vi "rsscope_core_global.vi"() -> ()   [LabVIEW 2018] (continued)
TrigA, TrigB, TrigR\r\n\nRemote-control command(s):\nTRIGger<m>:RFFE:ERRor:USEQuence"}, {"Level"=4, "Class Only"=FALSE, "Identifier"="RSSCOPE_ATTR_PROTOCOL_RFFE_TRIGGER_ERROR_GAP", "Descriptive Name"="Protocol RFFE Trigger Error Gap", "Data Type"=3, "Command"="TRIG{Trigger}:RFFE:ERR:GAP", "Access"=2, "Range Table"="", "Read Callback"="", "Write Callback"="", "Supported Models"="", "Instrument Options"="K40", "Flags"=0, "Help"="Enables the trigger on a gap error.\n\nAvailable Repeated Capabilities:\nTrigger: TrigA, TrigB, TrigR\r\n\nRemote-control command(s):\nTRIGger<m>:RFFE:ERRor:GAP"}, {"Level"=4, "Class Only"=FALSE, "Identifier"="RSSCOPE_ATTR_PROTOCOL_RFFE_TRIGGER_ERROR_VERSION", "Descriptive Name"="Protocol RFFE Trigger Error Version", "Data Type"=3, "Command"="TRIG{Trigger}:RFFE:ERR:VERS", "Access"=2, "Range Table"="", "Read Callback"="", "Write Callback"="", "Supported Models"="", "Instrument Options"="K40", "Flags"=0, "Help"="Enables the trigger on RFFE version error.\n\nAvailable Repeated Capabilities:\nTrigger: TrigA, TrigB, TrigR\r\n\nRemote-control command(s):\nTRIGger<m>:RFFE:ERRor:VERSion"}, {"Level"=2, "Class Only"=TRUE, "Identifier"="", "Descriptive Name"="MDIO", "Data Type"=0, "Command"="", "Access"=0, "Range Table"="", "Read Callback"="", "Write Callback"="", "Supported Models"="", "Instrument Options"="", "Flags"=0, "Help"="Configures MDIO trigger, option K55."}, {"Level"=3, "Class Only"=FALSE, "Identifier"="RSSCOPE_ATTR_PROTOCOL_MDIO_TRIGGER_TYPE", "Descriptive Name"="Protocol MDIO Trigger Type", "Data Type"=0, "Command"="TRIG{Trigger}:MDIO:TYPE", "Access"=2, "Range Table"="rsscope_rngProtocolMDIOTriggerType", "Read Callback"="", "Write Callback"="", "Supported Models"="", "Instrument Options"="K55", "Flags"=0, "Help"="Selects the trigger type for MDIO analysis.\n\nAvailable Repeated Capabilities:\nTrigger: TrigA, TrigB, TrigR\r\n\nRemote-control command(s):\nTRIGger<m>:MDIO:TYPE"}, {"Level"=3, "Class Only"=FALSE, "Identifier"="RSSCOPE_ATTR_PROTOCOL_MDIO_TRIGGER_START_CODE", "Descriptive Name"="Protocol MDIO Trigger Start Code", "Data Type"=0, "Command"="TRIG{Trigger}:MDIO:ST", "Access"=2, "Range Table"="rsscope_rngProtocolMDIOTriggerStartCode", "Read Callback"="", "Write Callback"="", "Supported Models"="", "Instrument Options"="K55", "Flags"=0, "Help"="Selects the start of frame code of the frame pattern.\n\nAvailable Repeated Capabilities:\nTrigger: TrigA, TrigB, TrigR\r\n\nRemote-control command(s):\nTRIGger<m>:MDIO:ST"}, {"Level"=3, "Class Only"=FALSE, "Identifier"="RSSCOPE_ATTR_PROTOCOL_MDIO_TRIGGER_OPERATION_CODE", "Descriptive Name"="Protocol MDIO Trigger Operation Code", "Data Type"=0, "Command"="TRIG{Trigger}:MDIO:FRAM", "Access"=2, "Range Table"="rsscope_rngProtocolMDIOTriggerOperationCode", "Read Callback"="", "Write Callback"="", "Supported Models"="", "Instrument Options"="K55", "Flags"=0, "Help"="Selects the Type of Frame code (or OP code, OpCode, operation code).\n\nAvailable Repeated Capabilities:\nTrigger: TrigA, TrigB, TrigR\r\n\nRemote-control command(s):\nTRIGger<m>:MDIO:FRAMetype"}, {"Level"=3, "Class Only"=FALSE, "Identifier"="RSSCOPE_ATTR_PROTOCOL_MDIO_TRIGGER_PHYSICAL_PORT_ADDRESS", "Descriptive Name"="Protocol MDIO Trigger Physical Port Address", "Data Type"=2, "Command"="TRIG{Trigger}:MDIO:PHYS", "Access"=2, "Range Table"="", "Read Callback"="", "Write Callback"="", "Supported Models"="", "Instrument Options"="K55", "Flags"=0, "Help"="Sets the physical address (in Clause 22) or port address (in Clause 45) of the frame pattern (5 bits).\n\nAvailable Repeated Capabilities:\nTrigger: TrigA, TrigB, TrigR\r\n\nRemote-control command(s):\nTRIGger<m>:MDIO:PHYS"}, {"Level"=3, "Class Only"=FALSE, "Identifier"="RSSCOPE_ATTR_PROTOCOL_MDIO_TRIGGER_REGISTER_DEVICE_ADDRESS", "Descriptive Name"="Protocol MDIO Trigger Register Device Address", "Data Type"=2, "Command"="TRIG{Trigger}:MDIO:REGI", "Access"=2, "Range Table"="", "Read Callback"="", "Write Callback"="", "Supported Models"="", "Instrument Options"="K55", "Flags"=0, "Help"="Sets the register address (in Clause 22) or device address (in Clause 45) of the frame pattern (5 bits); available only in trigger type &apos;Data&apos;.\n\nAvailable Repeated Capabilities:\nTrigger: TrigA, TrigB, TrigR\r\n\nRemote-control command(s):\nTRIGger<m>:MDIO:REGI"}, {"Level"=3, "Class Only"=FALSE, "Identifier"="RSSCOPE_ATTR_PROTOCOL_MDIO_TRIGGER_DATA_ADDRESS_PATTERN", "Descriptive Name"="Protocol MDIO Trigger Data Address Pattern", "Data Type"=2, "Command"="TRIG{Trigger}:MDIO:DATA", "Access"=2, "Range Table"="", "Read Callback"="", "Write Callback"="", "Supported Models"="", "Instrument Options"="K55", "Flags"=0, "Help"="Defines the 16-bit payload data pattern (both in Clause 22 or Clause 45) or the address pattern (in Clause 45, only) to trigger for.\n\nAvailable Repeated Capabilities:\nTrigger: TrigA, TrigB, TrigR\r\n\nRemote-control command(s):\nTRIGger<m>:MDIO:DATA"}, {"Level"=2, "Class Only"=TRUE, "Identifier"="", "Descriptive Name"="Ethernet", "Data Type"=0, "Command"="", "Access"=0, "Range Table"="", "Read Callback"="", "Write Callback"="", "Supported Models"="", "Instrument Options"="", "Flags"=0, "Help"="Configures Ethernet trigger settings.\n\nAttributes in this class require option R&S RTO-K8."}, {"Level"=3, "Class Only"=FALSE, "Identifier"="RSSCOPE_ATTR_ETHERNET_TRIGGER_TYPE", "Descriptive Name"="Ethernet Trigger Type", "Data Type"=0, "Command"="TRIG{Trigger}:ETH:TYPE", "Access"=2, "Range Table"="RsScope_rngEthernetTriggerType", "Read Callback"="", "Write Callback"="", "Supported Models"="", "Instrument Options"="K8", "Flags"=0, "Help"="Sets the trigger type for Ethernet variant 10BASE-T.\n\nAvailable Repeated Capabilities:\nTrigger: TrigA, TrigB, TrigR\r\n\nRemote-control command(s):\nTRIGger<m>:ETHernet:TYPE"}, {"Level"=3, "Class Only"=FALSE, "Identifier"="RSSCOPE_ATTR_ETHERNET_TRIGGER_PATTERN", "Descriptive Name"="Ethernet Trigger Pattern", "Data Type"=2, "Command"="TRIG{Trigger}:ETH:PATT", "Access"=2, "Range Table"="", "Read Callback"="", "Write Callback"="", "Supported Models"="", "Instrument Options"="K8", "Flags"=0, "Help"="Specifies the bit pattern (or data) that is to be triggered.\n\nAvailable Repeated Capabilities:\nTrigger: TrigA, TrigB, TrigR\r\n\nRemote-control command(s):\nTRIGger<m>:ETHernet:PATTern"}, {"Level"=3, "Class Only"=FALSE, "Identifier"="RSSCOPE_ATTR_ETHERNET_TRIGGER_ERROR_CRC", "Descriptive Name"="Ethernet Trigger Error CRC", "Data Type"=3, "Command"="TRIG{Trigger}:ETH:ERR:CRC", "Access"=2, "Range Table"="", "Read Callback"="", "Write Callback"="", "Supported Models"="", "Instrument Options"="K8", "Flags"=0, "Help"="Enables the trigger on a mismatch of the cyclic redundancy check (CRC) value between the transmitting and receiving device.\n\nAvailable Repeated Capabilities:\nTrigger: TrigA, TrigB, TrigR\r\n\nRemote-control command(s):\nTRIGger<m>:ETHernet:ERRor:CRC"}, {"Level"=3, "Class Only"=FALSE, "Identifier"="RSSCOPE_ATTR_ETHERNET_TRIGGER_ERROR_LENGTH", "Descriptive Name"="Ethernet Trigger Error Length", "Data Type"=3, "Command"="TRIG{Trigger}:ETH:ERR:LENG", "Access"=2, "Range Table"="", "Read Callback"="", "Write Callback"="", "Supported Models"="", "Instrument Options"="K8", "Flags"=0, "Help"="Enables the trigger on an incorrect length of the sequence - when additional or missing bits are detected and the sequence of bits is not as expected.\n\nAvailable Repeated Capabilities:\nTrigger: TrigA, TrigB, TrigR\r\n\nRemote-control command(s):\nTRIGger<m>:ETHernet:ERRor:LENGth"}, {"Level"=3, "Class Only"=FALSE, "Identifier"="RSSCOPE_ATTR_ETHERNET_TRIGGER_ERROR_PREAMBLE", "Descriptive Name"="Ethernet Trigger Error Preamble", "Data Type"=3, "Command"="TRIG{Trigger}:ETH:ERR:PRE", "Access"=2, "Range Table"="", "Read Callback"="", "Write Callback"="", "Supported Models"="", "Instrument Options"="K8", "Flags"=0, "Help"="Enables the trigger on a frame with invalid preamble.\n\nAvailable Repeated Capabilities:\nTrigger: TrigA, TrigB, TrigR\r\n\nRemote-control command(s):\nTRIGger<m>:ETHernet:ERRor:PREamble"}, {"Level"=3, "Class Only"=TRUE, "Identifier"="", "Descriptive Name"="Frame", "Data Type"=0, "Command"="", "Access"=0, "Range Table"="", "Read Callback"="", "Write Callback"="", "Supported Models"="", "Instrument Options"="", "Flags"=0, "Help"="Configures Ethernet frame."}, {"Level"=4, "Class Only"=FALSE, "Identifier"="RSSCOPE_ATTR_ETHERNET_TRIGGER_FRAME_CRC_CONDITION", "Descriptive Name"="Ethernet Trigger Frame CRC Condition", "Data Type"=0, "Command"="TRIG{Trigger}:ETH:FRAM:CCON", "Access"=2, "Range Table"="RsScope_rngProtocolEthernetTriggerDataCondition", "Read Callback"="", "Write Callback"="", "Supported Models"="", "Instrument Options"="K8", "Flags"=0, "Help"="Sets the operator to trigger on a specific frame check sequence value.\n\nAvailable Repeated Capabilities:\nTrigger: TrigA, TrigB, TrigR\r\n\nRemote-control command(s):\nTRIGger<m>:ETHernet:FRAMe:CCONdition"}, {"Level"=4, "Class Only"=FALSE, "Identifier"="RSSCOPE_ATTR_ETHERNET_TRIGGER_FRAME_CRC_PATTERN_MIN", "Descriptive Name"="Ethernet Trigger Frame CRC Pattern Min", "Data Type"=2, "Command"="TRIG{Trigger}:ETH:FRAM:CMIN", "Access"=2, "Range Table"="", "Read Callback"="", "Write Callback"="", "Supported Models"="", "Instrument Options"="K8", "Flags"=0, "Help"="Specifies a CRC pattern, or sets the start value of a pattern range.\n\nAvailable Repeated Capabilities:\nTrigger: TrigA, TrigB, TrigR\r\n\nRemote-control command(s):\nTRIGger<m>:ETHernet:FRAMe:CMIN"}, {"Level"=4, "Class Only"=FALSE, "Identifier"="RSSCOPE_ATTR_ETHERNET_TRIGGER_FRAME_CRC_PATTERN_MAX", "Descriptive Name"="Ethernet Trigger Frame CRC Pattern Max", "Data Type"=2, "Command"="TRIG{Trigger}:ETH:FRAM:CMAX", "Access"=2, "Range Table"="", "Read Callback"="", "Write Callback"="", "Supported Models"="", "Instrument Options"="K8", "Flags"=0, "Help"="Sets the end value of the frame check sequence range.\n\nAvailable Repeated Capabilities:\nTrigger: TrigA, TrigB, TrigR\r\n\nRemote-control command(s):\nTRIGger<m>:ETHernet:FRAMe:CMAX"}, {"Level"=4, "Class Only"=FALSE, "Identifier"="RSSCOPE_ATTR_ETHERNET_TRIGGER_FRAME_DESTINATION_ADDRESS_CONDITION", "Descriptive Name"="Ethernet Trigger Frame Destination Address Condition", "Data Type"=0, "Command"="TRIG{Trigger}:ETH:FRAM:DCON", "Access"=2, "Range Table"="RsScope_rngProtocolEthernetTriggerDataCondition", "Read Callback"="", "Write Callback"="", "Supported Models"="", "Instrument Options"="K8", "Flags"=0, "Help"="Sets the destination address operator to trigger on a specific pattern or a range.\n\nAvailable Repeated Capabilities:\nTrigger: TrigA, TrigB, TrigR\r\n\nRemote-control command(s):\nTRIGger<m>:ETHernet:FRAMe:DCONdition"}, {"Level"=4, "Class Only"=FALSE, "Identifier"="RSSCOPE_ATTR_ETHERNET_TRIGGER_FRAME_DESTINATION_ADDRESS_PATTERN_MIN", "Descriptive Name"="Ethernet Trigger Frame Destination Address Pattern Min", "Data Type"=2, "Command"="TRIG{Trigger}:ETH:FRAM:DMIN", "Access"=2, "Range Table"="", "Read Callback"="", "Write Callback"="", "Supported Models"="", "Instrument Options"="K8", "Flags"=0, "Help"="Specifies a destination address pattern, or sets the start value of a pattern range.\n\nAvailable Repeated Capabilities:\nTrigger: TrigA, TrigB, TrigR\r\n\nRemote-control command(s):\nTRIGger<m>:ETHernet:FRAMe:DMIN"}, {"Level"=4, "Class Only"=FALSE, "Identifier"="RSSCOPE_ATTR_ETHERNET_TRIGGER_FRAME_DESTINATION_ADDRESS_PATTERN_MAX", "Descriptive Name"="Ethernet Trigger Frame Destination Address Pattern Max", "Data Type"=2, "Command"="TRIG{Trigger}:ETH:FRAM:DMAX", "Access"=2, "Range Table"="", "Read Callback"="", "Write Callback"="", "Supported Models"="", "Instrument Options"="K8", "Flags"=0, "Help"="Sets the end value of a destination address range.\n\nAvailable Repeated Capabilities:\nTrigger: TrigA, TrigB, TrigR\r\n\nRemote-control command(s):\nTRIGger<m>:ETHernet:FRAMe:DMAX"}, {"Level"=4, "Class Only"=FALSE, "Identifier"="RSSCOPE_ATTR_ETHERNET_TRIGGER_FRAME_SOURCE_ADDRESS_CONDITION", "Descriptive Name"="Ethernet Trigger Frame Source Address Condition", "Data Type"=0, "Command"="TRIG{Trigger}:ETH:FRAM:SCON", "Access"=2, "Range Table"="RsScope_rngProtocolEthernetTriggerDataCondition", "Read Callback"="", "Write Callback"="", "Supported Models"="", "Instrument Options"="K8", "Flags"=0, "Help"="Sets source address operator to trigger on a specific pattern or a range.\n\nAvailable Repeated Capabilities:\nTrigger: TrigA, TrigB, TrigR\r\n\nRemote-control command(s):\nTRIGger<m>:ETHernet:FRAMe:SCONdition"}, {"Level"=4, "Class Only"=FALSE, "Identifier"="RSSCOPE_ATTR_ETHERNET_TRIGGER_FRAME_SOURCE_ADDRESS_PATTERN_MIN", "Descriptive Name"="Ethernet Trigger Frame Source Address Pattern Min", "Data Type"=2, "Command"="TRIG{Trigger}:ETH:FRAM:SMIN", "Access"=2, "Range Table"="", "Read Callback"="", "Write Callback"="", "Supported Models"="", "Instrument Options"="K8", "Flags"=0, "Help"="Specifies a source address pattern, or sets the start value of a pattern range.\n\nAvailable Repeated Capabilities:\nTrigger: TrigA, TrigB, TrigR\r\n\nRemote-control command(s):\nTRIGger<m>:ETHernet:FRAMe:SMIN"}, {"Level"=4, "Class Only"=FALSE, "Identifier"="RSSCOPE_ATTR_ETHERNET_TRIGGER_FRAME_SOURCE_ADDRESS_PATTERN_MAX", "Descriptive Name"="Ethernet Trigger Frame Source Address Pattern Max", "Data Type"=2, "Command"="TRIG{Trigger}:ETH:FRAM:SMAX", "Access"=2, "Range Table"="", "Read Callback"="", "Write Callback"="", "Supported Models"="", "Instrument Options"="K8", "Flags"=0, "Help"="Sets the end value of a source address range.\n\nAvailable Repeated Capabilities:\nTrigger: TrigA, TrigB, TrigR\r\n\nRemote-control command(s):\nTRIGger<m>:ETHernet:FRAMe:SMAX"}, {"Level"=4, "Class Only"=FALSE, "Identifier"="RSSCOPE_ATTR_ETHERNET_TRIGGER_FRAME_TYPE_OPERATOR_CONDITION", "Descriptive Name"="Ethernet Trigger Frame Type Operator Condition", "Data Type"=0, "Command"="TRIG{Trigger}:ETH:FRAM:TCON", "Access"=2, "Range Table"="RsScope_rngProtocolEthernetTriggerDataCondition", "Read Callback"="", "Write Callback"="", "Supported Models"="", "Instrument Options"="K8", "Flags"=0, "Help"="Sets the type operator to trigger on a specific length/type value pattern or a range.\n\nAvailable Repeated Capabilities:\nTrigger: TrigA, TrigB, TrigR\r\n\nRemote-control command(s):\nTRIGger<m>:ETHernet:FRAMe:TCONdition"}, {"Level"=4, "Class Only"=FALSE, "Identifier"="RSSCOPE_ATTR_ETHERNET_TRIGGER_FRAME_TYPE_OPERATOR_PATTERN_MIN", "Descriptive Name"="Ethernet Trigger Frame Type Operator Pattern Min", "Data Type"=2, "Command"="TRIG{Trigger}:ETH:FRAM:TMIN", "Access"=2, "Range Table"="", "Read Callback"="", "Write Callback"="", "Supported Models"="", "Instrument Options"="K8", "Flags"=0, "Help"="Specifies a length/type value, or sets the start value of a pattern range.\n\nAvailable Repeated Capabilities:\nTrigger: TrigA, TrigB, TrigR\r\n\nRemote-control command(s):\nTRIGger<m>:ETHernet:FRAMe:TMIN"}, {"Level"=4, "Class Only"=FALSE, "Identifier"="RSSCOPE_ATTR_ETHERNET_TRIGGER_FRAME_TYPE_OPERATOR_PATTERN_MAX", "Descriptive Name"="Ethernet Trigger Frame Type Operator Pattern Max", "Data Type"=2, "Command"="TRIG{Trigger}:ETH:FRAM:TMAX", "Access"=2, "Range Table"="", "Read Callback"="", "Write Callback"="", "Supported Models"="", "Instrument Options"="K8", "Flags"=0, "Help"="Sets the end value of a length/type range.\n\nAvailable Repeated Capabilities:\nTrigger: TrigA, TrigB, TrigR\r\n\nRemote-control command(s):\nTRIGger<m>:ETHernet:FRAMe:TMAX"}, {"Level"=2, "Class Only"=TRUE, "Identifier"="", "Descriptive Name"="USB", "Data Type"=0, "Command"="", "Access"=0, "Range Table"="", "Read Callback"="", "Write Callback"="", "Supported Models"="", "Instrument Options"="", "Flags"=0, "Help"="Configures USB trigger settings."}, {"Level"=3, "Class Only"=FALSE, "Identifier"="RSSCOPE_ATTR_PROTOCOL_USB_TRIGGER_TYPE", "Descriptive Name"="Protocol USB Trigger Type", "Data Type"=0, "Command"="TRIG{Trigger}:USB:TYPE", "Access"=2, "Range Table"="rsscope_rngProtocolUSBTriggerType", "Read Callback"="", "Write Callback"="", "Supported Models"="", "Instrument Options"="K60", "Flags"=0, "Help"="Selects the trigger type for USB analysis. The available trigger types depend on the activated USB protocol type.\n\nAvailable Repeated Capabilities:\nTrigger: TrigA, TrigB, TrigR\r\n\nRemote-control command(s):\nTRIGger<m>:USB:TYPE"}, {"Level"=3, "Class Only"=FALSE, "Identifier"="RSSCOPE_ATTR_PROTOCOL_USB_TRIGGER_TOKEN", "Descriptive Name"="Protocol USB Trigger Token", "Data Type"=0, "Command"="TRIG{Trigger}:USB:TOK", "Access"=2, "Range Table"="rsscope_rngProtocolUSBTriggerToken", "Read Callback"="", "Write Callback"="", "Supported Models"="", "Instrument Options"="K60", "Flags"=0, "Help"="Sets the trigger to one out of four different token types: Out, In, Start of Frame, or Setup.\n\nAvailable Repeated Capabilities:\nTrigger: TrigA, TrigB, TrigR\r\n\nRemote-control command(s):\nTRIGger<m>:USB:TOKen"}, {"Level"=3, "Class Only"=FALSE, "Identifier"="RSSCOPE_ATTR_PROTOCOL_USB_TRIGGER_DATA_TYPE", "Descriptive Name"="Protocol USB Trigger Data Type", "Data Type"=0, "Command"="TRIG{Trigger}:USB:DATA", "Access"=2, "Range Table"="rsscope_rngProtocolUSBTriggerDataType", "Read Callback"="", "Write Callback"="", "Supported Models"="", "Instrument Options"="K60", "Flags"=0, "Help"="Sets the trigger to one out of four different payload data types: DATA0, DATA1, DATA2, or MDATA.\n\nAvailable Repeated Capabilities:\nTrigger: TrigA, TrigB, TrigR\r\n\nRemote-control command(s):\nTRIGger<m>:USB:DATA"}, {"Level"=3, "Class Only"=FALSE, "Identifier"="RSSCOPE_ATTR_PROTOCOL_USB_TRIGGER_HANDSHAKE", "Descriptive Name"="Protocol USB Trigger Handshake", "Data Type"=0, "Command"="TRIG{Trigger}:USB:HAND", "Access"=2, "Range Table"="rsscope_rngProtocolUSBTriggerHandshake", "Read Callback"="", "Write Callback"="", "Supported Models"="", "Instrument Options"="", "Flags"=0, "Help"="Sets the trigger to one out of four different handshake types: acknowledgment, non-acknowledgment, stall, or no response.\n\nAvailable Repeated Capabilities:\nTrigger: TrigA, TrigB, TrigR\r\n\nRemote-control command(s):\nTRIGger<m>:USB:HAND"}, {"Level"=3, "Class Only"=FALSE, "Identifier"="RSSCOPE_ATTR_PROTOCOL_USB_TRIGGER_SPECIAL_PID", "Descriptive Name"="Protocol USB Trigger Special PID", "Data Type"=0, "Command"="TRIG{Trigger}:USB:SPEC", "Access"=2, "Range Table"="rsscope_rngProtocolUSBTriggerSpecialPID", "Read Callback"="", "Write Callback"="", "Supported Models"="", "Instrument Options"="K60", "Flags"=0, "Help"="Sets the trigger to one out of four different Special PID types: Preamble, Error, Split, or Ping.\n\nAvailable Repeated Capabilities:\nTrigger: TrigA, TrigB, TrigR\r\n\nRemote-control command(s):\nTRIGger<m>:USB:SPEC"}, {"Level"=3, "Class Only"=FALSE, "Identifier"="RSSCOPE_ATTR_PROTOCOL_USB_TRIGGER_ERROR_CONDITION", "Descriptive Name"="Protocol USB Trigger Error Condition", "Data Type"=0, "Command"="TRIG{Trigger}:USB:ERRC", "Access"=2, "Range Table"="rsscope_rngProtocolUSBTriggerErrorCondition", "Read Callback"="", "Write Callback"="", "Supported Models"="", "Instrument Options"="K60", "Flags"=0, "Help"="Sets the trigger to one of the following eight error condition types: PID error, CRC5 error, CRC16 error, Bitstuffing error, unexpected PID error, SE1 error, or Glitching error, as well as Any of these errors.\n\nAvailable Repeated Capabilities:\nTrigger: TrigA, TrigB, TrigR\r\n\nRemote-control command(s):\nTRIGger<m>:USB:ERRC"}, {"Level"=3, "Class Only"=FALSE, "Identifier"="RSSCOPE_ATTR_PROTOCOL_USB_TRIGGER_PID_ERROR_CHECK", "Descriptive Name"="Protocol USB Trigger PID Error Check", "Data Type"=3, "Command"="TRIG{Trigger}:USB:WPID", "Access"=2, "Range Table"="", "Read Callback"="", "Write Callback"="", "Supported Models"="", "Instrument Options"="K60", "Flags"=0, "Help"="Defines, whether the packet ID error check shall be activated or not.\n\nAvailable Repeated Capabilities:\nTrigger: TrigA, TrigB, TrigR\r\n\nRemote-control command(s):\nTRIGger<m>:USB:WPID"}, {"Level"=3, "Class Only"=TRUE, "Identifier"="", "Descriptive Name"="End Point Check", "Data Type"=0, "Command"="", "Access"=0, "Range Table"="", "Read Callback"="", "Write Callback"="", "Supported Models"="", "Instrument Options"="", "Flags"=0, "Help"="Defines, whether an endpoint check that meets specific conditions is executed or not."}, {"Level"=4, "Class Only"=FALSE, "Identifier"="RSSCOPE_ATTR_PROTOCOL_USB_TRIGGER_END_POINT_CHECK", "Descriptive Name"="Protocol USB Trigger End Point Check", "Data Type"=3, "Command"="TRIG{Trigger}:USB:WEND", "Access"=2, "Range Table"="", "Read Callback"="", "Write Callback"="", "Supported Models"="", "Instrument Options"="K60", "Flags"=0, "Help"="Defines, whether the endpoint check shall be activated or not.\n\nAvailable Repeated Capabilities:\nTrigger: TrigA, TrigB, TrigR\r\n\nRemote-control command(s):\nTRIGger<m>:USB:WEND"}, {"Level"=4, "Class Only"=FALSE, "Identifier"="RSSCOPE_ATTR_PROTOCOL_USB_TRIGGER_END_POINT_CHECK_CONDITION", "Descriptive Name"="Protocol USB Trigger End Point Check Condition", "Data Type"=0, "Command"="TRIG{Trigger}:USB:ECON", "Access"=2, "Range Table"="rsscope_rngProtocolTriggerCondition", "Read Callback"="", "Write Callback"="", "Supported Models"="", "Instrument Options"="K60", "Flags"=0, "Help"="Sets the operator to set a specific endpoint or an endpoint range.\n\nAvailable Repeated Capabilities:\nTrigger: TrigA, TrigB, TrigR\r\n\nRemote-control command(s):\nTRIGger<m>:USB:ECONdition"}, {"Level"=4, "Class Only"=FALSE, "Identifier"="RSSCOPE_ATTR_PROTOCOL_USB_TRIGGER_END_POINT_CHECK_MIN", "Descriptive Name"="Protocol USB Trigger End Point Check Min", "Data Type"=2, "Command"="TRIG{Trigger}:USB:EMIN", "Access"=2, "Range Table"="", "Read Callback"="", "Write Callback"="", "Supported Models"="", "Instrument Options"="K60", "Flags"=0, "Help"="Specifies the endpoint, or sets the start value of an endpoint range.\n\nAvailable Repeated Capabilities:\nTrigger: TrigA, TrigB, TrigR\r\n\nRemote-control command(s):\nTRIGger<m>:USB:EMIN"}, {"Level"=4, "Class Only"=FALSE, "Identifier"="RSSCOPE_ATTR_PROTOCOL_USB_TRIGGER_END_POINT_CHECK_MAX", "Descriptive Name"="Protocol USB Trigger End Point Check Max", "Data Type"=2, "Command"="TRIG{Trigger}:USB:EMAX", "Access"=2, "Range Table"="", "Read Callback"="", "Write Callback"="", "Supported Models"="", "Instrument Options"="K60", "Flags"=0, "Help"="Sets the end value of an endpoint range if the corresponding condition is set to &apos;In range&apos; and &apos;Out of range&apos;.\n\nAvailable Repeated Capabilities:\nTrigger: TrigA, TrigB, TrigR\r\n\nRemote-control command(s):\nTRIGger<m>:USB:EMAX"}, {"Level"=3, "Class Only"=TRUE, "Identifier"="", "Descriptive Name"="Address Check", "Data Type"=0, "Command"="", "Access"=0, "Range Table"="", "Read Callback"="", "Write Callback"="", "Supported Models"="", "Instrument Options"="", "Flags"=0, "Help"="Defines, whether an address check that meets specific conditions is executed or not."}, {"Level"=4, "Class Only"=FALSE, "Identifier"="RSSCOPE_ATTR_PROTOCOL_USB_TRIGGER_ADDRESS_CHECK", "Descriptive Name"="Protocol USB Trigger Address Check", "Data Type"=3, "Command"="TRIG{Trigger}:USB:WADD", "Access"=2, "Range Table"="", "Read Callback"="", "Write Callback"="", "Supported Models"="", "Instrument Options"="K60", "Flags"=0, "Help"="Defines, whether the address check shall be activated or not.\n\nAvailable Repeated Capabilities:\nTrigger: TrigA, TrigB, TrigR\r\n\nRemote-control command(s):\nTRIGger<m>:USB:WADD"}, {"Level"=4, "Class Only"=FALSE, "Identifier"="RSSCOPE_ATTR_PROTOCOL_USB_TRIGGER_ADDRESS_CHECK_CONDITION", "Descriptive Name"="Protocol USB Trigger Address Check Condition", "Data Type"=0, "Command"="TRIG{Trigger}:USB:ACON", "Access"=2, "Range Table"="rsscope_rngProtocolTriggerCondition", "Read Callback"="", "Write Callback"="", "Supported Models"="", "Instrument Options"="K60", "Flags"=0, "Help"="Sets the operator to set a specific endpoint or an endpoint range.\n\nAvailable Repeated Capabilities:\nTrigger: TrigA, TrigB, TrigR\r\n\nRemote-control command(s):\nTRIGger<m>:USB:ACONdition"}, {"Level"=4, "Class Only"=FALSE, "Identifier"="RSSCOPE_ATTR_PROTOCOL_USB_TRIGGER_ADDRESS_CHECK_MIN", "Descriptive Name"="Protocol USB Trigger Address Check Min", "Data Type"=2, "Command"="TRIG{Trigger}:USB:AMIN", "Access"=2, "Range Table"="", "Read Callback"="", "Write Callback"="", "Supported Models"="", "Instrument Options"="K60", "Flags"=0, "Help"="Specifies the address, or sets the start value of an address range.\n\nAvailable Repeated Capabilities:\nTrigger: TrigA, TrigB, TrigR\r\n\nRemote-control command(s):\nTRIGger<m>:USB:AMIN"}, {"Level"=4, "Class Only"=FALSE, "Identifier"="RSSCOPE_ATTR_PROTOCOL_USB_TRIGGER_ADDRESS_CHECK_MAX", "Descriptive Name"="Protocol USB Trigger Address Check Max", "Data Type"=2, "Command"="TRIG{Trigger}:USB:AMAX", "Access"=2, "Range Table"="", "Read Callback"="", "Write Callback"="", "Supported Models"="", "Instrument Options"="K60", "Flags"=0, "Help"="Sets the end value of an address range if the corresponding condition is set to &apos;In range&apos; and &apos;Out of range&apos;.\n\nAvailable Repeated Capabilities:\nTrigger: TrigA, TrigB, TrigR\r\n\nRemote-control command(s):\nTRIGger<m>:USB:AMAX"}, {"Level"=3, "Class Only"=TRUE, "Identifier"="", "Descriptive Name"="Payload Check", "Data Type"=0, "Command"="", "Access"=0, "Range Table"="", "Read Callback"="", "Write Callback"="", "Supported Models"="", "Instrument Options"="", "Flags"=0, "Help"="Defines, whether a payload check that meets specific conditions is executed or not."}, {"Level"=4, "Class Only"=FALSE, "Identifier"="RSSCOPE_ATTR_PROTOCOL_USB_TRIGGER_PAYLOAD_CHECK", "Descriptive Name"="Protocol USB Trigger Payload Check", "Data Type"=3, "Command"="TRIG{Trigger}:USB:WPAY", "Access"=2, "Range Table"="", "Read Callback"="", "Write Callback"="", "Supported Models"="", "Instrument Options"="K60", "Flags"=0, "Help"="Defines, whether the payload data check shall be activated or not.\n\nAvailable Repeated Capabilities:\nTrigger: TrigA, TrigB, TrigR\r\n\nRemote-control command(s):\nTRIGger<m>:USB:WPAY"}, {"Level"=4, "Class Only"=FALSE, "Identifier"="RSSCOPE_ATTR_PROTOCOL_USB_TRIGGER_PAYLOAD_CHECK_CONDITION", "Descriptive Name"="Protocol USB Trigger Payload Check Condition", "Data Type"=0, "Command"="TRIG{Trigger}:USB:DPOP", "Access"=2, "Range Table"="rsscope_rngProtocolUSBPayloadCondition", "Read Callback"="", "Write Callback"="", "Supported Models"="", "Instrument Options"="K60", "Flags"=0, "Help"="Sets the operator (any or equal) for the payload data index position.\n\nAvailable Repeated Capabilities:\nTrigger: TrigA, TrigB, TrigR\r\n\nRemote-control command(s):\nTRIGger<m>:USB:DPOPerator"}, {"Level"=4, "Class Only"=FALSE, "Identifier"="RSSCOPE_ATTR_PROTOCOL_USB_TRIGGER_PAYLOAD_CHECK_POSITION", "Descriptive Name"="Protocol USB Trigger Payload Check Position", "Data Type"=0, "Command"="TRIG{Trigger}:USB:DPOS", "Access"=2, "Range Table"="rsscope_rngProtocolUSBPayloadPosition", "Read Callback"="", "Write Callback"="", "Supported Models"="", "Instrument Options"="K60", "Flags"=0, "Help"="Specifies the position within a payload data packet, in which a special data pattern is to be searched.\n\nAvailable Repeated Capabilities:\nTrigger: TrigA, TrigB, TrigR\r\n\nRemote-control command(s):\nTRIGger<m>:USB:DPOSition"}, {"Level"=4, "Class Only"=FALSE, "Identifier"="RSSCOPE_ATTR_PROTOCOL_USB_TRIGGER_PAYLOAD_CHECK_DATA_CONDITION", "Descriptive Name"="Protocol USB Trigger Payload Check Data Condition", "Data Type"=0, "Command"="TRIG{Trigger}:USB:DCON", "Access"=2, "Range Table"="rsscope_rngNqEq", "Read Callback"="", "Write Callback"="", "Supported Models"="", "Instrument Options"="K60", "Flags"=0, "Help"="Sets the operator (equal or unequal) to set a specific payload data pattern.\n\nAvailable Repeated Capabilities:\nTrigger: TrigA, TrigB, TrigR\r\n\nRemote-control command(s):\nTRIGger<m>:USB:DCONdition"}, {"Level"=4, "Class Only"=FALSE, "Identifier"="RSSCOPE_ATTR_PROTOCOL_USB_TRIGGER_PAYLOAD_CHECK_PATTERN", "Descriptive Name"="Protocol USB Trigger Payload Check Pattern", "Data Type"=2, "Command"="TRIG{Trigger}:USB:PATT", "Access"=2, "Range Table"="", "Read Callback"="", "Write Callback"="", "Supported Models"="", "Instrument Options"="K60", "Flags"=0, "Help"="Specifies the payload data pattern that is to be searched.\n\nAvailable Repeated Capabilities:\nTrigger: TrigA, TrigB, TrigR\r\n\nRemote-control command(s):\nTRIGger<m>:USB:PATT"}, {"Level"=3, "Class Only"=TRUE, "Identifier"="", "Descriptive Name"="Frame Check", "Data Type"=0, "Command"="", "Access"=0, "Range Table"="", "Read Callback"="", "Write Callback"="", "Supported Models"="", "Instrument Options"="", "Flags"=0, "Help"="Defines, whether a frame number check that meets specific conditions is executed or not."}, {"Level"=4, "Class Only"=FALSE, "Identifier"="RSSCOPE_ATTR_PROTOCOL_USB_TRIGGER_FRAME_CHECK", "Descriptive Name"="Protocol USB Trigger Frame Check", "Data Type"=3, "Command"="TRIG{Trigger}:USB:WFRN", "Access"=2, "Range Table"="", "Read Callback"="", "Write Callback"="", "Supported Models"="", "Instrument Options"="K60", "Flags"=0, "Help"="Defines, whether the frame number check shall be activated or not.\n\nAvailable Repeated Capabilities:\nTrigger: TrigA, TrigB, TrigR\r\n\nRemote-control command(s):\nTRIGger<m>:USB:WFRN"}, {"Level"=4, "Class Only"=FALSE, "Identifier"="RSSCOPE_ATTR_PROTOCOL_USB_TRIGGER_FRAME_CHECK_CONDITION", "Descriptive Name"="Protocol USB Trigger Frame Check Condition", "Data Type"=0, "Command"="TRIG{Trigger}:USB:FCON", "Access"=2, "Range Table"="rsscope_rngProtocolTriggerCondition", "Read Callback"="", "Write Callback"="", "Supported Models"="", "Instrument Options"="K60", "Flags"=0, "Help"="Sets the operator to set a specific frame number or a frame number range.\n\nAvailable Repeated Capabilities:\nTrigger: TrigA, TrigB, TrigR\r\n\nRemote-control command(s):\nTRIGger<m>:USB:FCONdition"}, {"Level"=4, "Class Only"=FALSE, "Identifier"="RSSCOPE_ATTR_PROTOCOL_USB_TRIGGER_FRAME_CHECK_MIN", "Descriptive Name"="Protocol USB Trigger Frame Check Min", "Data Type"=2, "Command"="TRIG{Trigger}:USB:FMIN", "Access"=2, "Range Table"="", "Read Callback"="", "Write Callback"="", "Supported Models"="", "Instrument Options"="K60", "Flags"=0, "Help"="Specifies the frame number, or sets the start value of a frame number range.\n\nAvailable Repeated Capabilities:\nTrigger: TrigA, TrigB, TrigR\r\n\nRemote-control command(s):\nTRIGger<m>:USB:FMIN"}, {"Level"=4, "Class Only"=FALSE, "Identifier"="RSSCOPE_ATTR_PROTOCOL_USB_TRIGGER_FRAME_CHECK_MAX", "Descriptive Name"="Protocol USB Trigger Frame Check Max", "Data Type"=2, "Command"="TRIG{Trigger}:USB:FMAX", "Access"=2, "Range Table"="", "Read Callback"="", "Write Callback"="", "Supported Models"="", "Instrument Options"="K60", "Flags"=0, "Help"="Sets the end value of a frame number range if the corresponding condition is set to &apos;In range&apos; and &apos;Out of range&apos;.\n\nAvailable Repeated Capabilities:\nTrigger: TrigA, TrigB, TrigR\r\n\nRemote-control command(s):\nTRIGger<m>:USB:FMAX"}, {"Level"=3, "Class Only"=TRUE, "Identifier"="", "Descriptive Name"="SC Check", "Data Type"=0, "Command"="", "Access"=0, "Range Table"="", "Read Callback"="", "Write Callback"="", "Supported Models"="", "Instrument Options"="", "Flags"=0, "Help"="Defines, whether a Start / Complete SPLIT transaction check is executed or not."}, {"Level"=4, "Class Only"=FALSE, "Identifier"="RSSCOPE_ATTR_PROTOCOL_USB_TRIGGER_SC_CHECK", "Descriptive Name"="Protocol USB Trigger SC Check", "Data Type"=3, "Command"="TRIG{Trigger}:USB:WSTC", "Access"=2, "Range Table"="", "Read Callback"="", "Write Callback"="", "Supported Models"="", "Instrument Options"="K60", "Flags"=0, "Help"="Defines, whether the frame number check shall be activated or not.\n\nAvailable Repeated Capabilities:\nTrigger: TrigA, TrigB, TrigR\r\n\nRemote-control command(s):\nTRIGger<m>:USB:WSTC"}, {"Level"=4, "Class Only"=FALSE, "Identifier"="RSSCOPE_ATTR_PROTOCOL_USB_TRIGGER_SC_CHECK_START_COMPLETE", "Descriptive Name"="Protocol USB Trigger SC Check Start Complete", "Data Type"=0, "Command"="TRIG{Trigger}:USB:STCO", "Access"=2, "Range Table"="rsscope_rngProtocolUSBSCCheckStartComplete", "Read Callback"="", "Write Callback"="", "Supported Models"="", "Instrument Options"="K60", "Flags"=0, "Help"="Sets the trigger to a specific start-split or complete-split transaction endpoint.\n\nAvailable Repeated Capabilities:\nTrigger: TrigA, TrigB, TrigR\r\n\nRemote-control command(s):\nTRIGger<m>:USB:STCO"}, {"Level"=3, "Class Only"=TRUE, "Identifier"="", "Descriptive Name"="Port Check", "Data Type"=0, "Command"="", "Access"=0, "Range Table"="", "Read Callback"="", "Write Callback"="", "Supported Models"="", "Instrument Options"="", "Flags"=0, "Help"="Defines, whether a frame number check that meets specific conditions is executed or not."}, {"Level"=4, "Class Only"=FALSE, "Identifier"="RSSCOPE_ATTR_PROTOCOL_USB_TRIGGER_PORT_CHECK", "Descriptive Name"="Protocol USB Trigger Port Check", "Data Type"=3, "Command"="TRIG{Trigger}:USB:WPOR", "Access"=2, "Range Table"="", "Read Callback"="", "Write Callback"="", "Supported Models"="", "Instrument Options"="K60", "Flags"=0, "Help"="Defines, whether the port check shall be activated or not.\n\nAvailable Repeated Capabilities:\nTrigger: TrigA, TrigB, TrigR\r\n\nRemote-control command(s):\nTRIGger<m>:USB:WPOR"}, {"Level"=4, "Class Only"=FALSE, "Identifier"="RSSCOPE_ATTR_PROTOCOL_USB_TRIGGER_PORT_CHECK_CONDITION", "Descriptive Name"="Protocol USB Trigger Port Check Condition", "Data Type"=0, "Command"="TRIG{Trigger}:USB:PCON", "Access"=2, "Range Table"="rsscope_rngProtocolTriggerCondition", "Read Callback"="", "Write Callback"="", "Supported Models"="", "Instrument Options"="K60", "Flags"=0, "Help"="Sets the operator to set a specific port number or a port number range.\n\nAvailable Repeated Capabilities:\nTrigger: TrigA, TrigB, TrigR\r\n\nRemote-control command(s):\nTRIGger<m>:USB:PCONdition"}, {"Level"=4, "Class Only"=FALSE, "Identifier"="RSSCOPE_ATTR_PROTOCOL_USB_TRIGGER_PORT_CHECK_MIN", "Descriptive Name"="Protocol USB Trigger Port Check Min", "Data Type"=2, "Command"="TRIG{Trigger}:USB:PMIN", "Access"=2, "Range Table"="", "Read Callback"="", "Write Callback"="", "Supported Models"="", "Instrument Options"="K60", "Flags"=0, "Help"="Specifies the port number, or sets the start value of a port number range.\n\nAvailable Repeated Capabilities:\nTrigger: TrigA, TrigB, TrigR\r\n\nRemote-control command(s):\nTRIGger<m>:USB:PMIN"}, {"Level"=4, "Class Only"=FALSE, "Identifier"="RSSCOPE_ATTR_PROTOCOL_USB_TRIGGER_PORT_CHECK_MAX", "Descriptive Name"="Protocol USB Trigger Port Check Max", "Data Type"=2, "Command"="TRIG{Trigger}:USB:PMAX", "Access"=2, "Range Table"="", "Read Callback"="", "Write Callback"="", "Supported Models"="", "Instrument Options"="K60", "Flags"=0, "Help"="Sets the end value of a port number range if the corresponding condition is set to &apos;In range&apos; and &apos;Out of range&apos;.\n\nAvailable Repeated Capabilities:\nTrigger: TrigA, TrigB, TrigR\r\n\nRemote-control command(s):\nTRIGger<m>:USB:PMAX"}, {"Level"=3, "Class Only"=TRUE, "Identifier"="", "Descriptive Name"="SEU Check", "Data Type"=0, "Command"="", "Access"=0, "Range Table"="", "Read Callback"="", "Write Callback"="", "Supported Models"="", "Instrument Options"="", "Flags"=0, "Help"="Defines, whether an SEU check that meets specific conditions is executed or not. S and E represent the Start and End of a start-split transaction, U represents the reserved/Unused bit of a complete-split transaction. Permissible binary SEU values are 00, 01, 10, and 11."}, {"Level"=4, "Class Only"=FALSE, "Identifier"="RSSCOPE_ATTR_PROTOCOL_USB_TRIGGER_SEU_CHECK", "Descriptive Name"="Protocol USB Trigger SEU Check", "Data Type"=3, "Command"="TRIG{Trigger}:USB:WSEU", "Access"=2, "Range Table"="", "Read Callback"="", "Write Callback"="", "Supported Models"="", "Instrument Options"="K60", "Flags"=0, "Help"="Defines, whether the SEU check shall be activated or not.\n\nAvailable Repeated Capabilities:\nTrigger: TrigA, TrigB, TrigR\r\n\nRemote-control command(s):\nTRIGger<m>:USB:WSEU"}, {"Level"=4, "Class Only"=FALSE, "Identifier"="RSSCOPE_ATTR_PROTOCOL_USB_TRIGGER_SEU_CHECK_CONDITION", "Descriptive Name"="Protocol USB Trigger SEU Check Condition", "Data Type"=0, "Command"="TRIG{Trigger}:USB:SCON", "Access"=2, "Range Table"="rsscope_rngProtocolTriggerCondition", "Read Callback"="", "Write Callback"="", "Supported Models"="", "Instrument Options"="K60", "Flags"=0, "Help"="Sets the operator to set a specific SEU or an SEU range.\n\nAvailable Repeated Capabilities:\nTrigger: TrigA, TrigB, TrigR\r\n\nRemote-control command(s):\nTRIGger<m>:USB:SCONdition"}, {"Level"=4, "Class Only"=FALSE, "Identifier"="RSSCOPE_ATTR_PROTOCOL_USB_TRIGGER_SEU_CHECK_MIN", "Descriptive Name"="Protocol USB Trigger SEU Check Min", "Data Type"=2, "Command"="TRIG{Trigger}:USB:SMIN", "Access"=2, "Range Table"="", "Read Callback"="", "Write Callback"="", "Supported Models"="", "Instrument Options"="K60", "Flags"=0, "Help"="Specifies the SEU, or sets the start value of an SEU range.\n\nAvailable Repeated Capabilities:\nTrigger: TrigA, TrigB, TrigR\r\n\nRemote-control command(s):\nTRIGger<m>:USB:SMIN"}, {"Level"=4, "Class Only"=FALSE, "Identifier"="RSSCOPE_ATTR_PROTOCOL_USB_TRIGGER_SEU_CHECK_MAX", "Descriptive Name"="Protocol USB Trigger SEU Check Max", "Data Type"=2, "Command"="TRIG{Trigger}:USB:SMAX", "Access"=2, "Range Table"="", "Read Callback"="", "Write Callback"="", "Supported Models"="", "Instrument Options"="K60", "Flags"=0, "Help"="Sets the end value of an SEU range if the corresponding condition is set to &apos;In range&apos; and &apos;Out of range&apos;.\n\nAvailable Repeated Capabilities:\nTrigger: TrigA, TrigB, TrigR\r\n\nRemote-control command(s):\nTRIGger<m>:USB:SMAX"}, {"Level"=3, "Class Only"=TRUE, "Identifier"="", "Descriptive Name"="ET Check", "Data Type"=0, "Command"="", "Access"=0, "Range Table"="", "Read Callback"="", "Write Callback"="", "Supported Models"="", "Instrument Options"="", "Flags"=0, "Help"="Defines, whether an Endpoint Type (ET) check that meets specific conditions is executed or not."}, {"Level"=4, "Class Only"=FALSE, "Identifier"="RSSCOPE_ATTR_PROTOCOL_USB_TRIGGER_ET_CHECK", "Descriptive Name"="Protocol USB Trigger ET Check", "Data Type"=3, "Command"="TRIG{Trigger}:USB:WETC", "Access"=2, "Range Table"="", "Read Callback"="", "Write Callback"="", "Supported Models"="", "Instrument Options"="K60", "Flags"=0, "Help"="Defines, whether the Endpoint Type (ET) check shall be activated or not.\n\nAvailable Repeated Capabilities:\nTrigger: TrigA, TrigB, TrigR\r\n\nRemote-control command(s):\nTRIGger<m>:USB:WETCheck"}, {"Level"=4, "Class Only"=FALSE, "Identifier"="RSSCOPE_ATTR_PROTOCOL_USB_TRIGGER_ET_CHECK_CONDITION", "Descriptive Name"="Protocol USB Trigger ET Check Condition", "Data Type"=0, "Command"="TRIG{Trigger}:USB:TCON", "Access"=2, "Range Table"="rsscope_rngProtocolTriggerCondition", "Read Callback"="", "Write Callback"="", "Supported Models"="", "Instrument Options"="K60", "Flags"=0, "Help"="Sets the operator to set a specific endpoint type (ET) or an ET range.\n\nAvailable Repeated Capabilities:\nTrigger: TrigA, TrigB, TrigR\r\n\nRemote-control command(s):\nTRIGger<m>:USB:TCONdition"}, {"Level"=4, "Class Only"=FALSE, "Identifier"="RSSCOPE_ATTR_PROTOCOL_USB_TRIGGER_ET_CHECK_MIN", "Descriptive Name"="Protocol USB Trigger ET Check Min", "Data Type"=2, "Command"="TRIG{Trigger}:USB:TMIN", "Access"=2, "Range Table"="", "Read Callback"="", "Write Callback"="", "Supported Models"="", "Instrument Options"="K60", "Flags"=0, "Help"="Specifies the endpoint type, or sets the start value of an endpoint type range.\n\nAvailable Repeated Capabilities:\nTrigger: TrigA, TrigB, TrigR\r\n\nRemote-control command(s):\nTRIGger<m>:USB:TMIN"}, {"Level"=4, "Class Only"=FALSE, "Identifier"="RSSCOPE_ATTR_PROTOCOL_USB_TRIGGER_ET_CHECK_MAX", "Descriptive 
